vi "MyIP (SubVI).vi"(8 "error in (no error)":errorcluster, 11 "IPArray":u32[](array[numeric]) format="%x") -> (0 "error out":errorcluster, 3 "Sel_IP_hex":u32)   [LabVIEW 2017]
panel:
  in  "Используемый сетевой интерфейс":u16(ring) items=["169.254.82.115", "192.168.1.197"]
  in  "Sel":bool
  in  "IpArrayStr":string[](array[string])
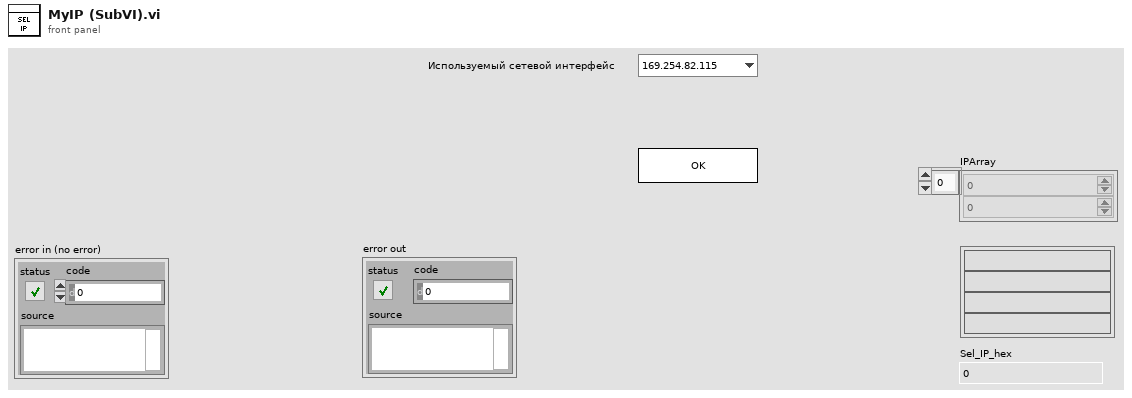
[diagram p1: front panel]
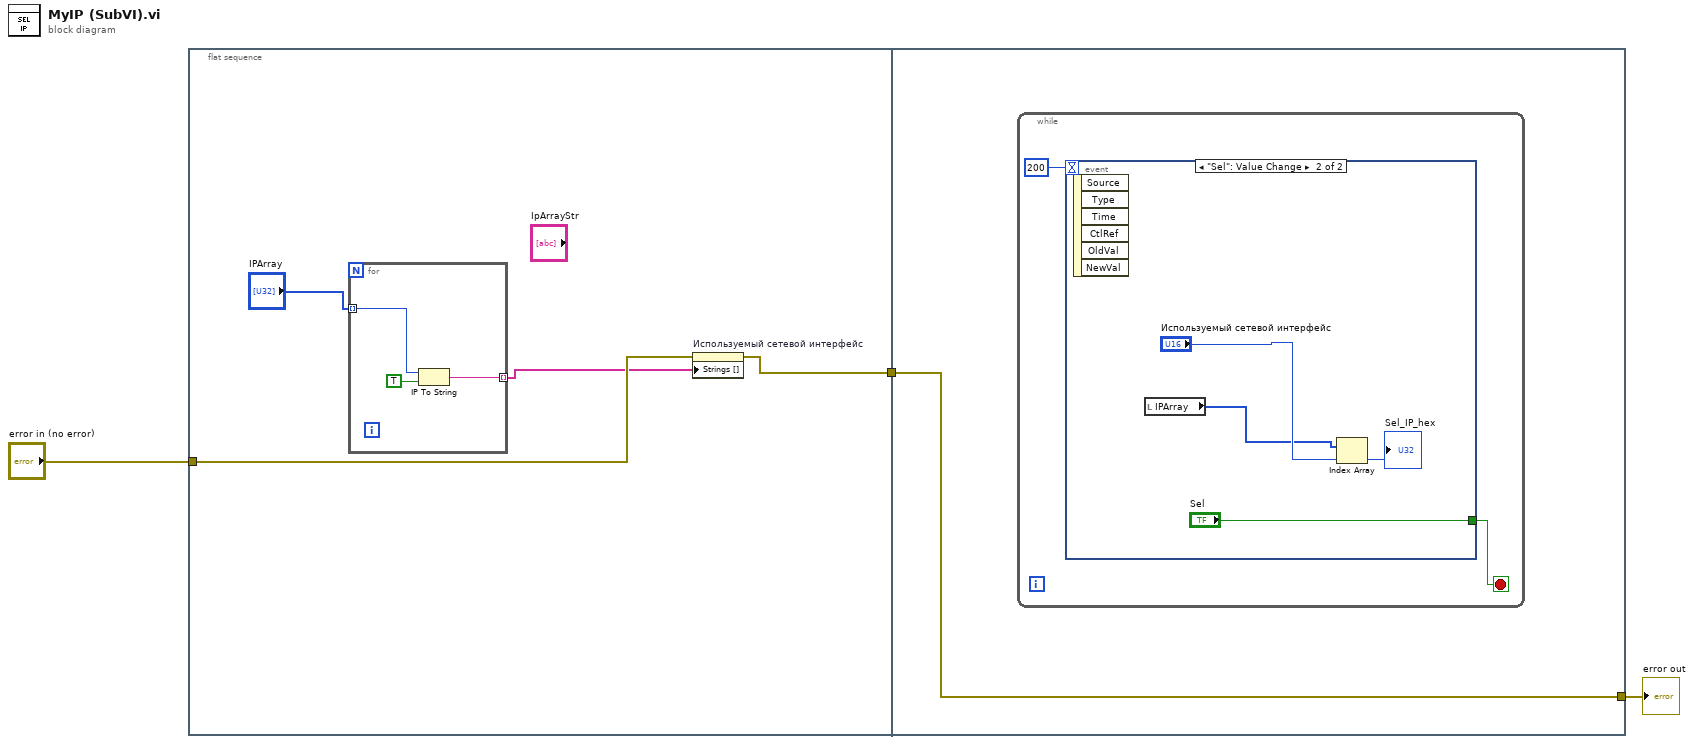
[diagram p0: block diagram]
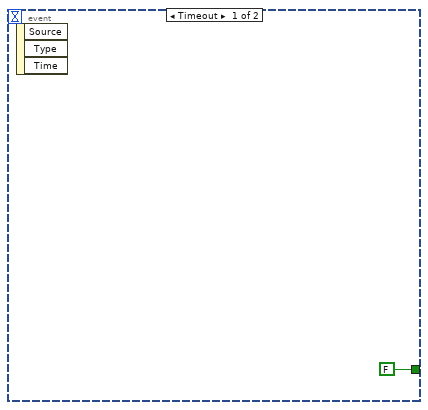
[diagram p2: hidden frame]
diagram:
  n1 = flat-sequence {
    tunnel: "error in (no error)" -> [w7]
    tunnel: [w6] -> w2
    tunnel: [w11] -> w1
    tunnel: w2 -> [w11]
    frame #0 {
      n2 = for {
        tunnel: "IPArray" -> [w9] mode=indexing
        tunnel: [w8] -> w4 mode=indexing
        n3 = IP To String(1:TRUE ("dot notation? (F)"), 2:w9) -> (0:w8:string)
      }
      n4 = property on="Используемый сетевой интерфейс" class="Ring (strict)"(error in=w7, "Strings []"=w4) -> (error out=w6:errorcluster)  [unwired: 1 in, 1 out]
    }
    frame #1 {
      n5 = while {
        stop <- w13 stop-if-true
        n6 = event shown="[1] \"Sel\": Value Change" {
          selector: _ -> [_ _]
          dyn-events: _ -> [_ _]
          timeout: 200 -> [_ _]
          tunnel: [FALSE ("Sel") "Sel"] -> w13
          event Timeout {
            n7 = event-data() -> ()  [unwired: 1 in, 3 out]
          }
          event "Sel": Value Change {
            n8 = event-data() -> ()  [unwired: 1 in, 6 out]
            n9 = local read "IPArray"() -> (w15:u32[])
            n10 = Index Array(array=w15, index="Используемый сетевой интерфейс") -> (element=→"Sel_IP_hex":u32)
          }
        }
      }
    }
  }
  "error out" <- w1
